vi "Apply Output.vi"(8 "error in":errorcluster, 11 "6512 in":refnum<class "6512.lvclass">) -> (0 "error out":errorcluster, 3 "6512 out":refnum<class "6512.lvclass">)   [LabVIEW 2019, in "6512.lvlib" / "6512.lvclass"]
uses:
  Library/6512.lvclass
  C:/Users/Public/Documents/Development/builds/Instruments/DigitalOut.lvlibp/Library/DigitalOut.lvclass
  builds/Instruments/DigitalOut.lvlibp/Accessors/Read Bank.vi
  builds/Instruments/DigitalOut.lvlibp/Accessors/Read Position.vi
  builds/Instruments/DigitalOut.lvlibp/Accessors/Read Value.vi
  builds/Instruments/DigitalOut.lvlibp/Accessors/Read Output State.vi
  builds/Instruments/DigitalOut.lvlibp/Accessors/Write Output State.vi
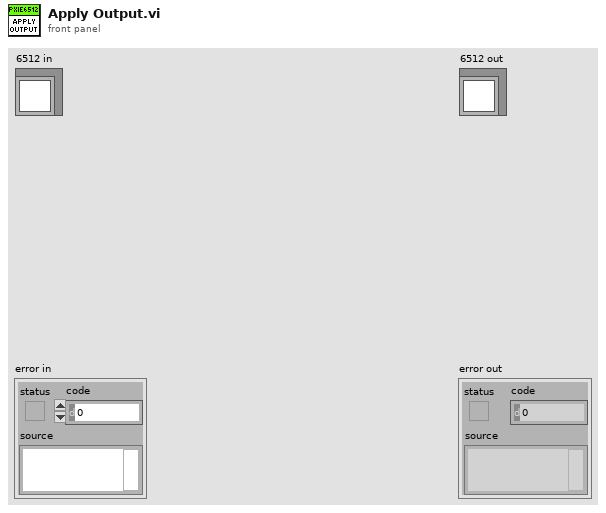
[diagram p1: front panel]
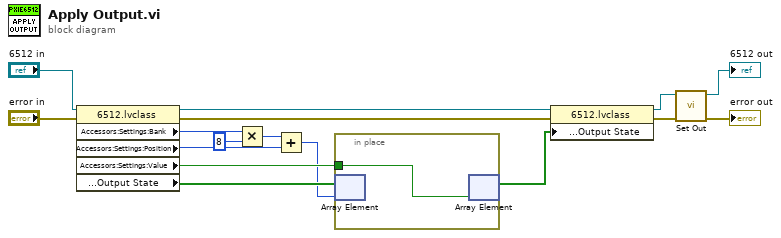
[diagram p0: block diagram]
diagram:
  n1 = property class="6512.lvclass"(reference="6512 in", error in="error in") -> (reference out=w7:refnum<class "6512.lvclass">, error out=w6:errorcluster, "Accessors:Settings:Bank"=w14:u32, "Accessors:Settings:Position"=w12:u32, "Accessors:Settings:Value"=w9:bool, "Accessors:Settings:Output State"=w10:bool[])
  n2 = Multiply(x=w14, y=u32 8) -> (x*y=w13:u32)
  n3 = Add(x=w13, y=w12) -> (x+y=w8:u32)
  n4 = in-place {
    in-place-border: w9 -> [w17]
    n5 = in-place-array #1(w10, w8) -> ()  [unwired: 1 out]
    n6 = in-place-array #1(w17) -> (w5:bool[])  [unwired: 1 out]
  }
  n7 = property class="6512.lvclass"(reference=w7, error in=w6, "Accessors:Settings:Output State"=w5) -> (reference out=w1:refnum<class "6512.lvclass">, error out=w4:errorcluster)
  n8 = call-dynamic "Set Out.vi"("error in"=w4, "6512 in"=w1) -> ("error out"=→"error out":errorcluster, "6512 out"=→"6512 out":refnum<class "6512.lvclass">)  [unwired: 8 in]
